vi "DependenciesUI.vi"() -> ()   [LabVIEW 2015, in "Dependencies.lvclass"]
uses:
  Dependencies.lvclass
  <vilib>/NI/Configuration Framework/Node/NodeRef.ctl
  <vilib>/NI/Configuration Framework/Node/NISE_CEF_Node.lvclass
  <vilib>/NI/AMC/Message Queue.ctl
  <vilib>/NI/AMC/Message.ctl
  <vilib>/NI/Tools/Keyed Array/KeyedArray.ctl
  <vilib>/NI/Configuration Framework/Node/UserEventRef.ctl
  <vilib>/NI/Configuration Framework/Controls/EventCluster.ctl
  XML Controls/Dependencies Properties.ctl
  XML Controls/Path Cluster.ctl
  XML Controls/Supported Targets.ctl
  <vilib>/NI/AMC/Create Single Message.vi
  <vilib>/NI/AMC/Update Message Routing Info.vi
  <vilib>/NI/AMC/Send Message.vi
  <vilib>/NI/AMC/AMC.lvlib
  Configuration Tool.lvlib
  <vilib>/NI/Tools/Keyed Array/Tools_KeyedArray.lvlib
  <vilib>/NI/Configuration Framework/NISE_CEF_TreeControl.lvlib
  VeriStand Custom Device XML Parser.lvlib
panel:
  in  "Main UI Tab":enum32{"Dependencies", "Dependencies 2"}(tab)
  in  "Add New":bool
  in  "Multicolumn Listbox":i32(listbox)
  out "ForceDownload":bool
  in  "Version":string
  out "Supported Target":T1(ring)
  in  "Real Time System Destination":string
  in  "Host Path to Dependency":path
  out "All Dependencies Properties":T2[](array[typedef])
  in  "Host Path to ActionVI":path
  in  "user event":T5
  in  "main queue":T6
  in  "node ref":T7
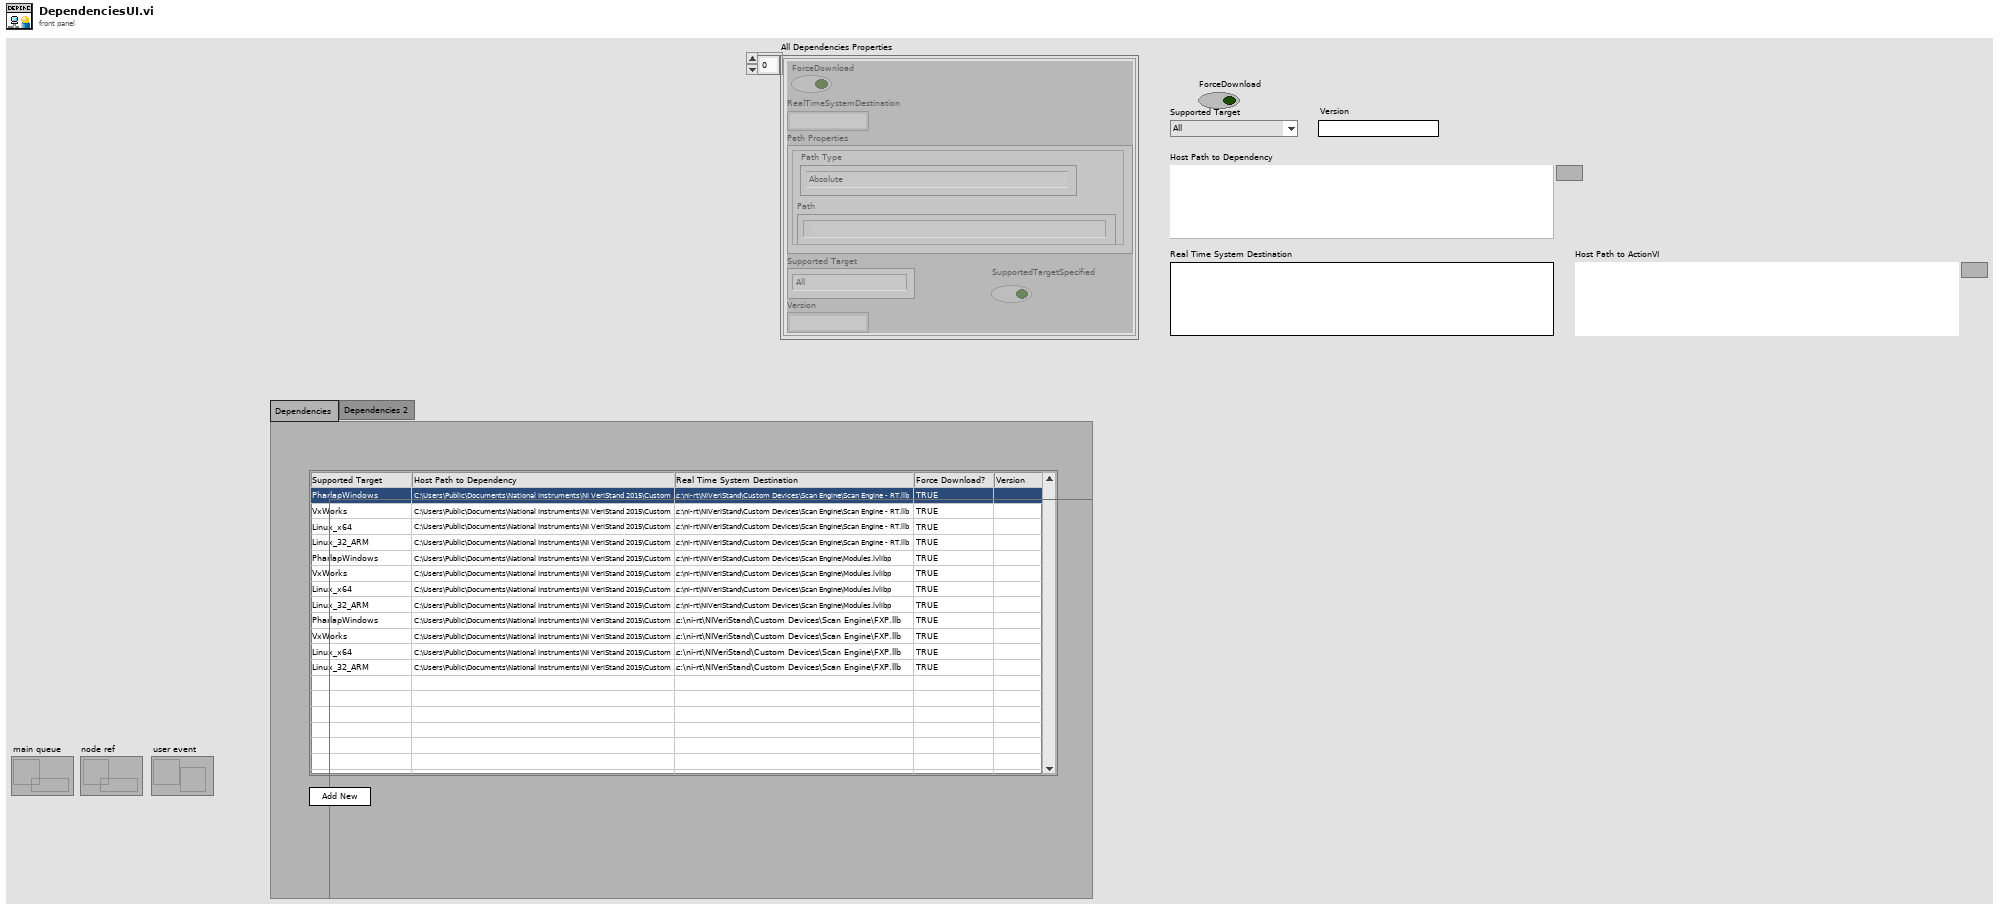
[diagram p1: front panel]
types:
  T1 = enum16{"All", "Pharlap", "VxWorks", "Windows", "Linux_32_ARM", "Linux_x64", "PharlapWindows", "PharlapVxWorks", "VxWorksWindows"}
  T2 = typedef "VeriStand Custom Device XML Parser.lvlib/Dependencies Properties.ctl" = cluster{"ForceDownload":bool, "RealTimeSystemDestination":string, "Path Properties":T3, "Supported Target":T4, "Version":string, "SupportedTargetSpecified":bool}
  T3 = typedef "VeriStand Custom Device XML Parser.lvlib/Path Cluster.ctl" = cluster{"Path":path, "Path Type":enum16{"Absolute", "To Base", "To Common Doc Dir", "To Application Data Dir"}}
  T4 = typedef "VeriStand Custom Device XML Parser.lvlib/Supported Targets.ctl" = enum16{"All", "Pharlap", "VxWorks", "Windows", "Linux_32_ARM", "Linux_x64", "PharlapWindows", "PharlapVxWorks", "VxWorksWindows"}
  T5 = typedef "NISE_CEF_Node.lvclass/UserEventRef.ctl" = refnum<user-event>
  T6 = typedef "AMC.lvlib/Message Queue.ctl" = refnum<queue>
  T7 = typedef "NISE_CEF_Node.lvclass/NodeRef.ctl" = refnum<data-value>
  T8 = enum16{"Absolute", "To Base", "To Common Doc Dir", "To Application Data Dir"}
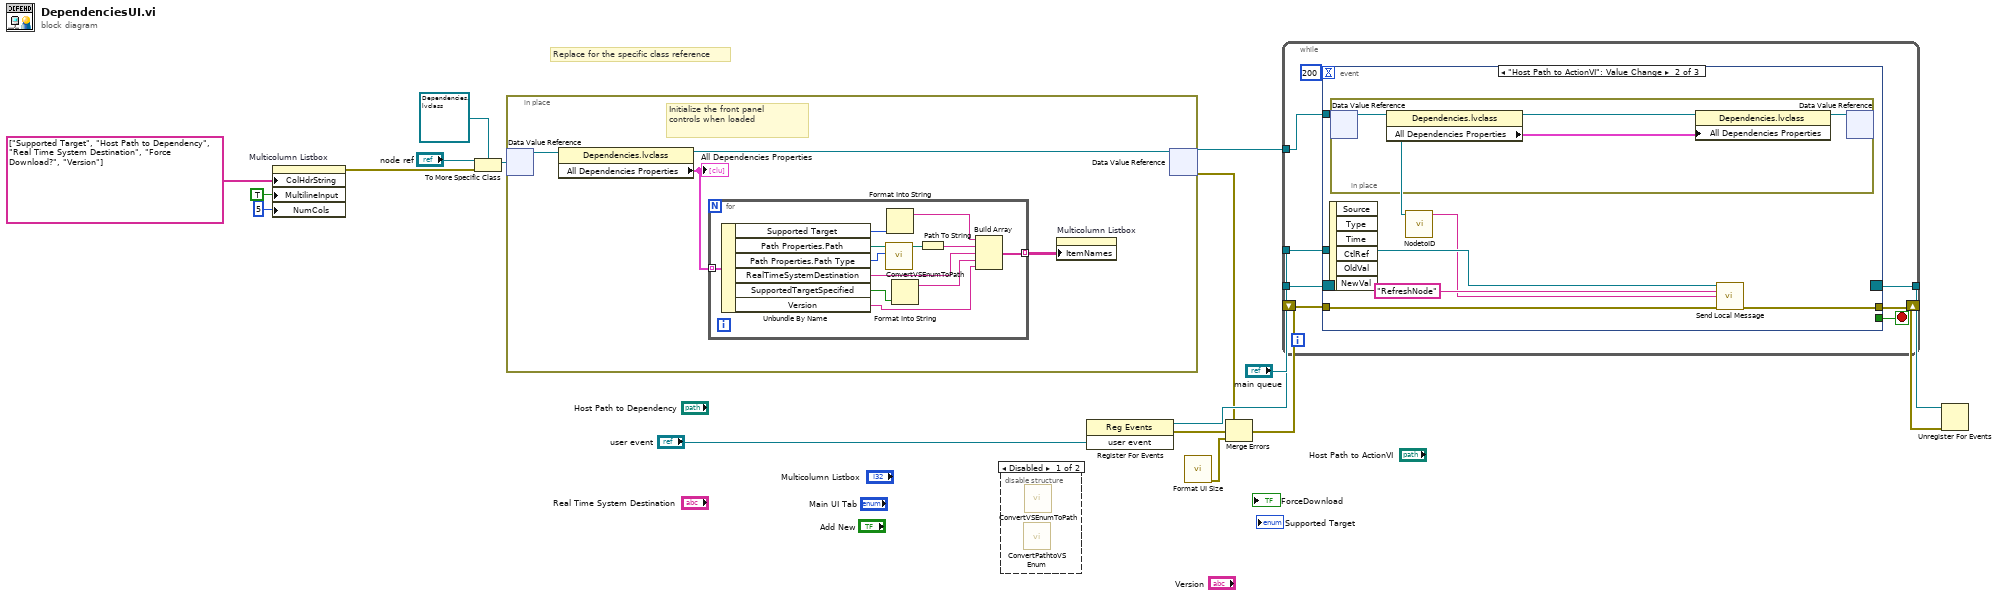
[diagram p0: block diagram]
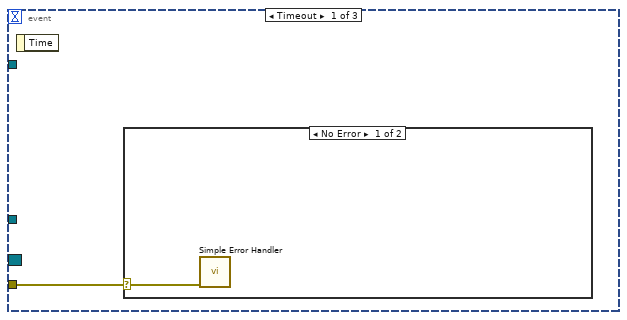
[diagram p3: hidden frame]
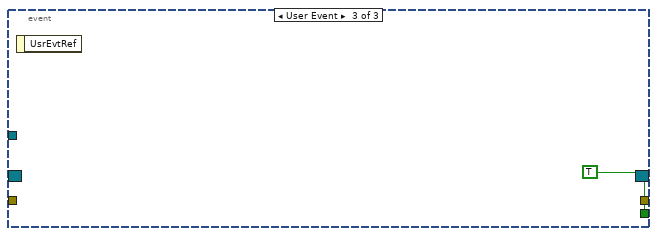
[diagram p5: hidden frame]
diagram:
  # "Replace for the specific class reference"
  n1 = property on="Multicolumn Listbox" class="MCListbox (strict)"("ColHdrString"=string[] ["Supported Target", "Host Path to Dependency", "Real Time System Destination", "Force Download?", "Version"] ("Column Header Strings[]"), "MultilineInput"=TRUE ("Multiple Line Input"), "NumCols"=u32 5 ("Number of Columns")) -> (error out=w2:errorcluster)  [unwired: 2 in, 1 out]
  n2 = To More Specific Class(target class=refnum<data-value> refnum ("data value reference"), reference="node ref", error in=w2) -> (specific class reference=w10:refnum<data-value>)  [unwired: 1 out]
  n3 = in-place {
    # "Initialize the front panel controls when loaded"
    n4 = in-place-dvr #1(w10) -> (w21:refnum<class "Dependencies.lvclass">)  [unwired: 1 out]
    n5 = property class="Dependencies.lvclass"(reference=w21) -> (reference out=w20:refnum<class "Dependencies.lvclass">, "All Dependencies Properties"=w19:T2[])  [unwired: 1 in, 1 out]
    "All Dependencies Properties" <- w19
    n6 = for {
      tunnel: w19 -> [w33] mode=indexing
      tunnel: [w25] -> w18 mode=indexing
      n7 = Unbundle By Name(w33) -> ("Supported Target"=w32:T4, "Path Properties.Path"=w31:path, "Path Properties.Path Type"=w30:T8, "RealTimeSystemDestination"=w26:string, "SupportedTargetSpecified"=w24:bool, "Version"=w22:string)
      n8 = call "ConvertVSEnumToPath.vi"("Source.Path Type"=w30, "Path In"=w31) -> ("appended path"=w29:path)  [unwired: 9 in]
      n9 = Format Into String(w32) -> (resulting string=w28:string)  [unwired: 3 in, 1 out]
      n10 = Format Into String(w24) -> (resulting string=w23:string)  [unwired: 3 in, 1 out]
      n11 = Path To String(path=w29) -> (string=w27:string)
      n12 = Build Array(w28, w27, w26, w23, w22) -> (w25:string[])
    }
    n13 = property on="Multicolumn Listbox" class="MCListbox (strict)"("ItemNames"=w18) -> ()  [unwired: 2 in, 2 out]
    n14 = in-place-dvr #1(w20) -> (w17:refnum<data-value>, w7:errorcluster)
  }
  n15 = disable-structure shown="Disabled" {
    frame Disabled {
      n16 = call "ConvertPathtoVSEnum.vi"() -> ()  [unwired: 10 in, 2 out]
      n17 = call "ConvertVSEnumToPath.vi"() -> ()  [unwired: 11 in, 1 out]
    }
    frame Enabled {
    }
  }
  n18 = register-events("user event") -> (reference out=w14:refnum<event-registration>, error out=w8:errorcluster)  [unwired: 2 in]
  n19 = call "Format UI Size.vi"() -> ("error out"=w1:errorcluster)  [unwired: 11 in]
  n20 = Merge Errors(w7, w8, w1) -> (w6:errorcluster)
  n21 = while {
    tunnel: w17 -> [w41]
    tunnel: "main queue" -> [w40]
    tunnel: w14 -> [w38]
    tunnel: [w37] -> w13
    shift-right: [w35] -> w12
    shift-left: w6 -> [w34]
    stop <- w36 stop-if-true
    n22 = event shown="[1] \"Host Path to ActionVI\": Value Change" {
      selector: w38 -> [_ _ _]
      dyn-events: [_ _ _] -> w37
      timeout: 200 -> [_ _ _]
      tunnel: w41 -> [_ w47 _]
      tunnel: w40 -> [_ w48 _]
      tunnel: [_ _ TRUE] -> w36
      tunnel: [_ w45 _] -> w35
      tunnel: w34 -> [w42 w44 _]
      event Timeout {
        n23 = event-data() -> ()  [unwired: 1 in, 1 out]
        n24 = case shown="No Error" w42 {
          selector: w42 -> [w43 _]
          frame No Error {
            n25 = call <vilib>:"Simple Error Handler.vi"("error in (no error)"=w43) -> ()  [unwired: 4 in, 5 out]
          }
          frame Error {
          }
        }
      }
      event "Host Path to ActionVI": Value Change {
        n26 = event-data() -> ()  [unwired: 1 in, 6 out]
        n27 = in-place {
          n28 = in-place-dvr #2(w47) -> (w52:refnum<class "Dependencies.lvclass">)  [unwired: 1 out]
          n29 = property class="Dependencies.lvclass"(reference=w52) -> (reference out=w51:refnum<class "Dependencies.lvclass">, "All Dependencies Properties"=w50:T2[])  [unwired: 1 in, 1 out]
          n30 = property class="Dependencies.lvclass"(reference=w51, "All Dependencies Properties"=w50) -> (reference out=w53:refnum<class "Dependencies.lvclass">)  [unwired: 1 in, 1 out]
          n31 = in-place-dvr #2(w53) -> ()  [unwired: 2 out]
        }
        n32 = call <vilib>:"NodetoID.vi"("node ref"=w47) -> ("ID"=w46:string)  [unwired: 9 in, 1 out]
        n33 = call <vilib>:"Send Local Message.vi"("message queue in"=w48, "message name"="RefreshNode" ("Message Name"), "message value"=w46, "error in"=w44) -> ("error out"=w45:errorcluster)  [unwired: 9 in, 2 out]
      }
      event User Event {
        n34 = event-data() -> ()  [unwired: 1 in, 1 out]
      }
    }
  }
  n35 = Unregister For Events(event registration refnum=w13, error in=w12) -> ()  [unwired: 1 out]
